vi "Start AsyncRepeatSum LowLevel.vi"(8 "error in":errorcluster, 9 "B":i32, 10 "A":i32, 11 "LVUserEventCallBackRef":refnum<user-event>) -> (0 "error out":errorcluster, 2 "Handle":u64)   [LabVIEW 2016, in "DemoSkeleton.lvlib"]
uses:
  DemoSkeleton.lvlib
  skeleton_lv_event_lvrt.dll
  skeleton_lv_event_lv.dll
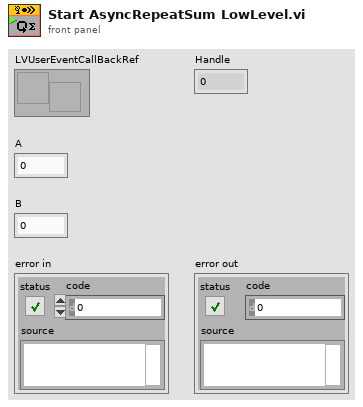
[diagram p1: front panel]
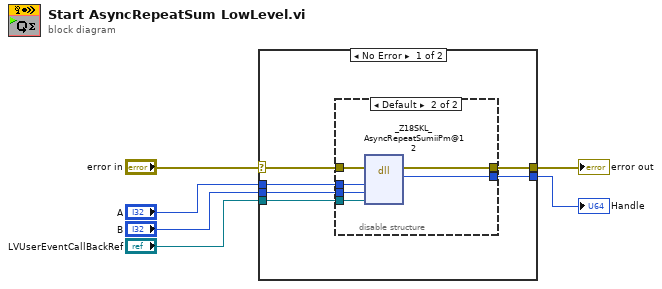
[diagram p0: block diagram]
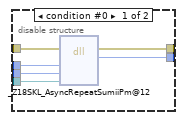
[diagram p2: hidden frame]
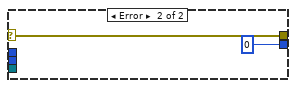
[diagram p3: hidden frame]
diagram:
  n1 = case shown="No Error" "error in" {
    selector: "error in" -> [w12 w26]
    tunnel: [w11 w26] -> w5
    tunnel: "A" -> [w10 _]
    tunnel: "B" -> [w9 _]
    tunnel: "LVUserEventCallBackRef" -> [w8 _]
    tunnel: [w7 u64 0 ("Handle")] -> w1
    frame No Error {
      n2 = disable-structure shown="Default" {
        disable-tunnel: [w15 w21] -> w7
        disable-tunnel: w12 -> [w18 w24]
        disable-tunnel: [w16 w22] -> w11
        disable-tunnel: w8 -> [w17 w23]
        disable-tunnel: w10 -> [w14 w20]
        disable-tunnel: w9 -> [w13 w19]
        frame condition #0 {
          n3 = dll-call lib="C:/Users/loic.wohleber/Desktop/PostLvUserEvent_Demo/Sources/LabVIEW/Library/DemoSkeleton/skeleton_lv_event_lvrt.dll" fn="_Z18SKL_AsyncRepeatSumiiPm@12" label="AsyncSum_RT"(error in=w18, "A"=w14, "B"=w13, "CallBackRefEvent"=w17) -> (error out=w16:errorcluster, "Handle"=w15:u64)  [unwired: 5 in, 1 out]
        }
        frame condition #1 (active) {
          n4 = dll-call lib="C:/Users/loic.wohleber/Desktop/PostLvUserEvent_Demo/Sources/LabVIEW/Library/DemoSkeleton/skeleton_lv_event_lv.dll" fn="_Z18SKL_AsyncRepeatSumiiPm@12" label="AsyncRepeatSum_LV"(error in=w24, "A"=w20, "B"=w19, "CallBackRefEvent"=w23) -> (error out=w22:errorcluster, "Handle"=w21:u64)  [unwired: 5 in, 1 out]
        }
      }
    }
    frame Error {
    }
  }
  "error out" <- w5
  "Handle" <- w1
